vi "simx Copy Paste Objects.vi"(0 "clientID":i32, 1 "newObjectCount":i32, 5 "objectHandles":i32, 7 "objectCount":i32, 9 "newObjectHandles":i32, 11 "error in (no error)":errorcluster, 12 "operationMode":i32) -> (3 "newObjectCount out":i32, 4 "function return":i32, 10 "newObjectHandles out":i32, 15 "error out":errorcluster)   [LabVIEW 2019, in "PXL_V-REP.lvlib"]
doc: "EXTAPI_DLLEXPORT simxInt simxCopyPasteObjects(simxInt clientID,const simxInt* objectHandles,simxInt objectCount,simxInt** newObjectHandles,simxInt* newObjectCount,simxInt operationMode);"
uses:
  PXL_V-REP.lvlib
  <userlib>/V-REP/remoteApi.dll
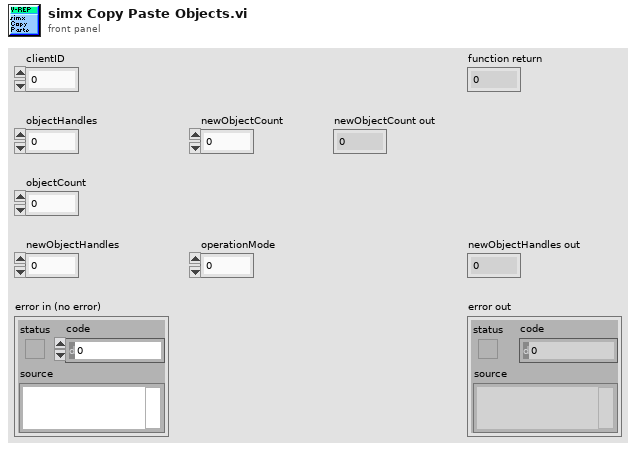
[diagram p1: front panel]
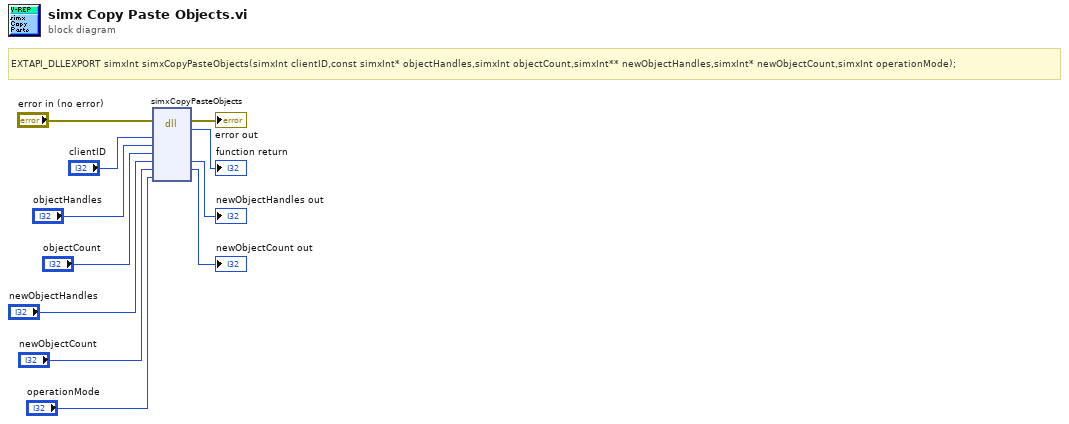
[diagram p0: block diagram]
diagram:
  # "EXTAPI_DLLEXPORT simxInt simxCopyPasteObjects(simxInt clientID,const simxInt* objectHandles,simxInt objectCount,simxInt** newObjectHandles,simxInt* newObjectCount,simxInt operationMode);"
  n1 = dll-call lib="C:/Program Files (x86)/National Instruments/LabVIEW 2019/user.lib/V-REP/remoteApi.*" fn="simxCopyPasteObjects"(error in="error in (no error)", "clientID"="clientID", "objectHandles"="objectHandles", "objectCount"="objectCount", "newObjectHandles"="newObjectHandles", "newObjectCount"="newObjectCount", "operationMode"="operationMode") -> (error out=→"error out":errorcluster, →"function return":i32, "newObjectHandles"=→"newObjectHandles out":i32, "newObjectCount"=→"newObjectCount out":i32)  [unwired: 6 in, 1 out]
